vi "last_index.vi"(4 "error in (no error)":errorcluster, 5 "py interface file":path, 6 "Request data":variant, 7 "Python session in":refnum<k35>) -> (0 "error out":errorcluster, 2 "Response data":variant, 3 "Python session out":refnum<k35>)   [LabVIEW 2022 SP3]
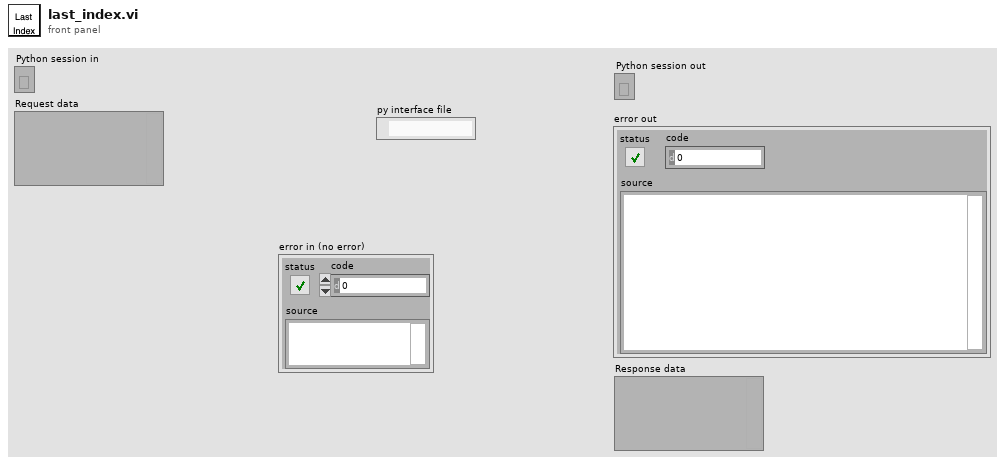
[diagram p1: front panel]
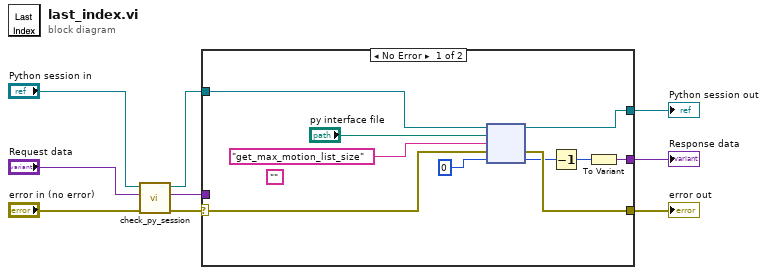
[diagram p0: block diagram]
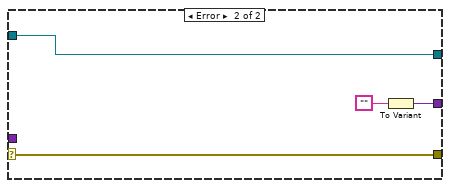
[diagram p2: hidden frame]
diagram:
  n1 = call "check_py_session.vi"("error in"="error in (no error)", "Request data"="Request data", "Python session in"="Python session in") -> ("error out"=w3:errorcluster, "Response data"=w4:variant, "Python session out"=w5:refnum<k35>)  [unwired: 2 in]
  n2 = case shown="No Error" w3 {
    selector: w3 -> [w10 w23]
    tunnel: w5 -> [w19 w22]
    tunnel: [w17 w22] -> w9
    tunnel: w4 -> [_ _]
    tunnel: [w16 w23] -> w2
    tunnel: [w15 w20] -> w1
    frame No Error {
      (unwired) ""
      n3 = node(w19, "py interface file", "get_max_motion_list_size" ("function name"), w10, 0) -> (w17:refnum<k35>, w16:errorcluster, w12:i32)  [unwired: 2 out]
      n4 = Decrement(x=w12) -> (x-1=w11:i32)
      n5 = To Variant(anything=w11) -> (Variant=w15:variant)
    }
    frame Error {
      n6 = To Variant(anything="") -> (Variant=w20:variant)
    }
  }
  "error out" <- w2
  "Python session out" <- w9
  "Response data" <- w1
